vi "write read back command.vi"(5 "Input Parameter":dbl format="%.2f", 6 "error in (no error)":errorcluster, 7 "Input Command":string, 8 "Timeout Limit":dbl format="%.2f", 9 "Port Number":refnum<visa-resource-name>) -> (0 "error out":errorcluster, 1 "Timeout":bool, 2 "Query Result":string, 3 "Status Byte":string)   [LabVIEW 2024]
uses:
  Serial Support VISA.llb/Serial Actions.ctl
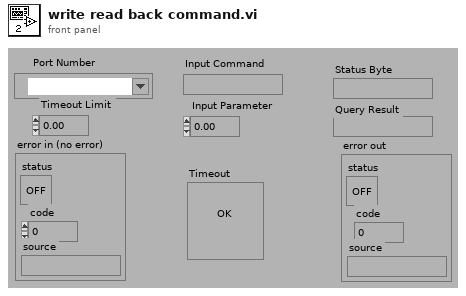
[diagram p1: front panel]
types:
  T1 = typedef "Serial Actions.ctl" = enum16{"Init", "Break", "Clear Buffer", "Write", "Read", "N Bytes", "Lock", "Unlock", "Close"}
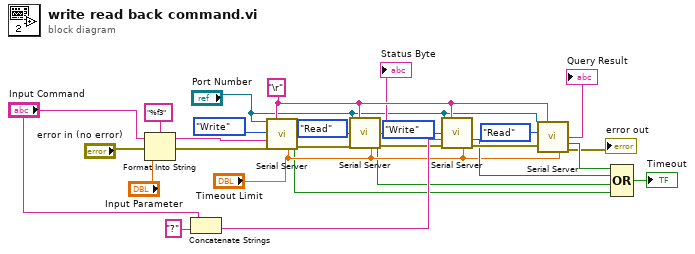
[diagram p0: block diagram]
diagram:
  w13 = "\r" ("EOT Chars (cr/lf)")
  n1 = Format Into String(format string="%f3", initial string="Input Command", error in="error in (no error)", "Input Parameter") -> (resulting string=w18:string, error out=w17:errorcluster)
  n2 = Concatenate Strings("Input Command", "?") -> (w15:string)
  n3 = call "Serial Server.vi"("VISA Resource Name"="Port Number", "EOT Chars (cr/lf)"=w13, "Action"=Serial_Actions."Write", "String To Send"=w18, "error in (no error)"=w17, "Timeout Limit(sec)"="Timeout Limit") -> ("Timeout"=w11:bool, "error out"=w8:errorcluster)  [unwired: 5 in, 3 out]
  n4 = call "Serial Server.vi"("VISA Resource Name"="Port Number", "EOT Chars (cr/lf)"=w13, "Action"=Serial_Actions."Read", "error in (no error)"=w8, "Timeout Limit(sec)"="Timeout Limit") -> ("Serial Read"=→"Status Byte":string, "Timeout"=w10:bool, "error out"=w7:errorcluster)  [unwired: 6 in, 2 out]
  n5 = call "Serial Server.vi"("VISA Resource Name"="Port Number", "EOT Chars (cr/lf)"=w13, "Action"=Serial_Actions."Write", "String To Send"=w15, "error in (no error)"=w7, "Timeout Limit(sec)"="Timeout Limit") -> ("Timeout"=w25:bool, "error out"=w26:errorcluster)  [unwired: 5 in, 3 out]
  n6 = call "Serial Server.vi"("VISA Resource Name"="Port Number", "EOT Chars (cr/lf)"=w13, "Action"=Serial_Actions."Read", "error in (no error)"=w26, "Timeout Limit(sec)"="Timeout Limit") -> ("Serial Read"=→"Query Result":string, "Timeout"=w24:bool, "error out"=→"error out":errorcluster)  [unwired: 6 in, 2 out]
  n7 = Compound Arithmetic op=OR(w24, w25, w10, w11) -> (→"Timeout":bool)
